vi "setArmAngles.vi"(1 "Enum":T1(ring), 2 "speed":i32, 3 "angle":i32) -> ()   [LabVIEW 2018]
uses:
  ARM angles.vi
panel:
  out "output variable":i32
  out "s2":i32
  out "s1":i32
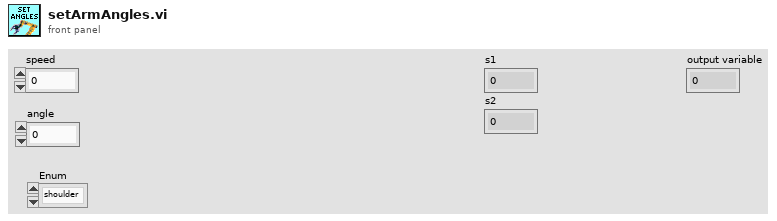
[diagram p1: front panel]
types:
  T1 = enum16{"shoulder", "elbow", "wrist", "base", "gripper"}
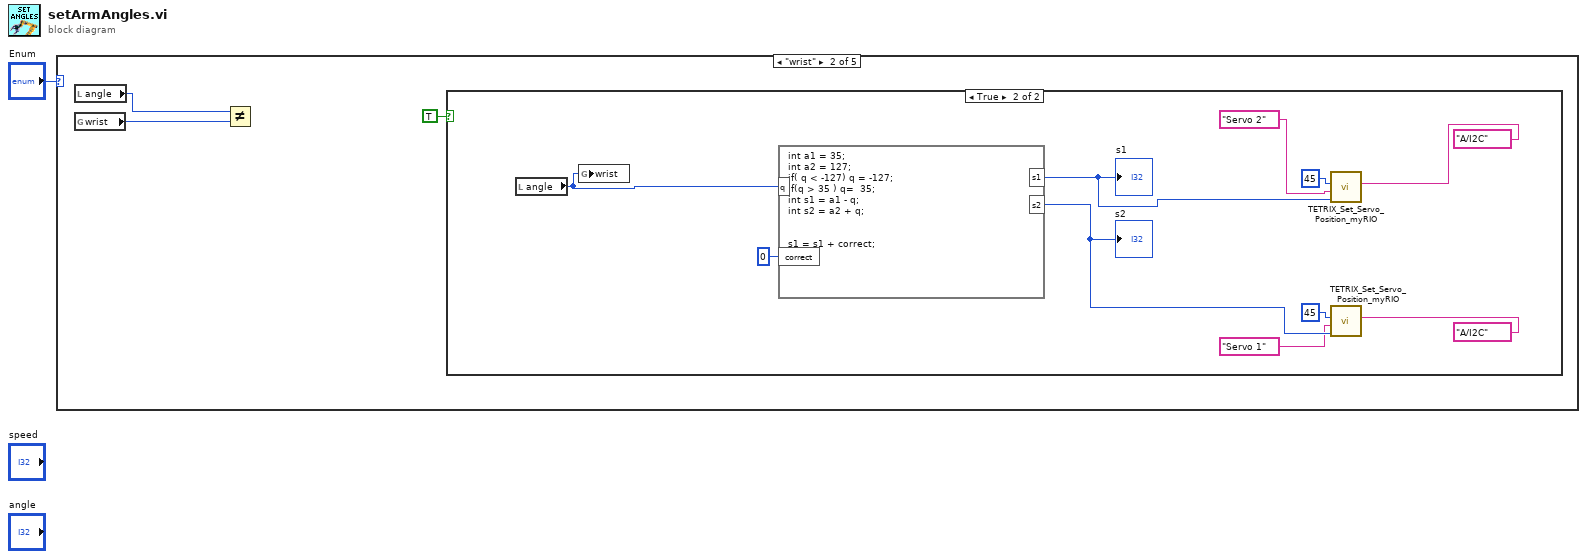
[diagram p0: block diagram]
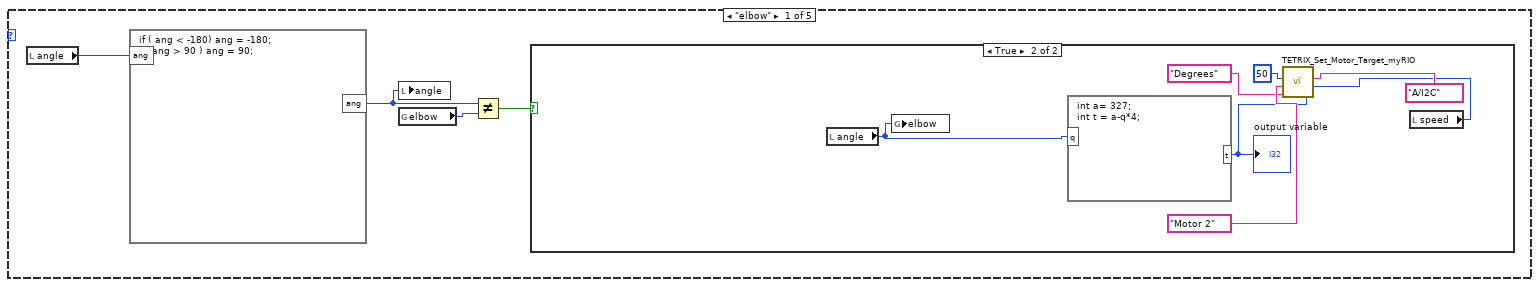
[diagram p2: hidden frame]
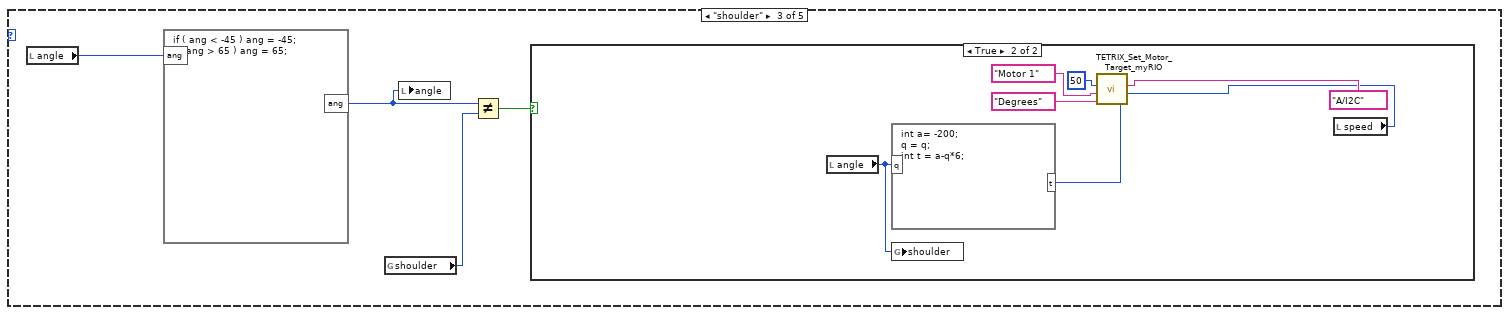
[diagram p5: hidden frame]
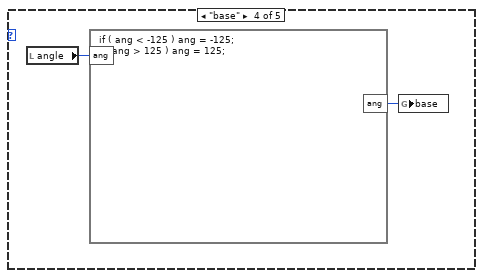
[diagram p7: hidden frame]
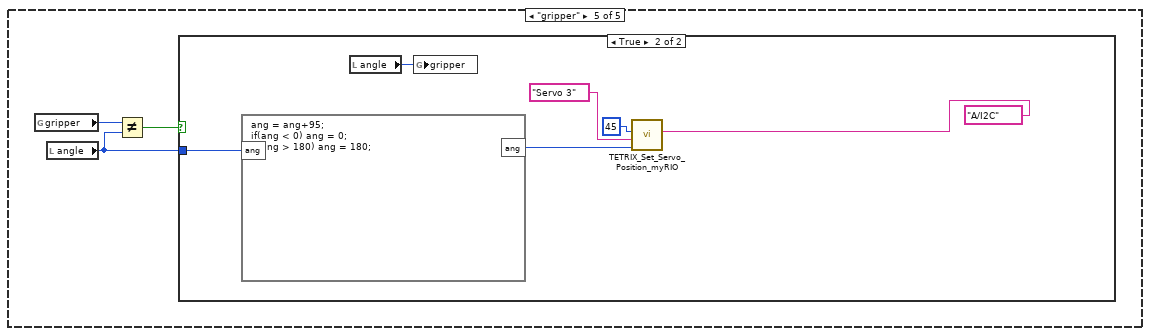
[diagram p8: hidden frame]
diagram:
  n1 = case shown="\"wrist\"" "Enum" {
    frame "elbow" {
      n2 = local read "angle"() -> (w3:i32)
      n3 = formula code="if ( ang < -180) ang = -180;\nif( ang > 90 ) ang = 90;"("ang"=w3) -> ("ang"=w2:i32)
      n4 = local write "angle"(w2) -> ()
      n5 = global read "ARM angles.vi" "elbow"() -> (w5:i32)
      n6 = Not Equal?(x=w2, y=w5) -> (x != y?=w4:bool)
      n7 = case shown="True" w4 {
        frame False {
        }
        frame True {
          n8 = local read "angle"() -> (w7:i32)
          n9 = global write "ARM angles.vi" "elbow"(w7) -> ()
          n10 = formula code="int a= 327;\nint t = a-q*4;"("q"=w7) -> ("t"=w6:i32)
          "output variable" <- w6
          n11 = local read "speed"() -> (w8:i32)
          n12 = call <vilib>:"TETRIX_Set_Motor_Target_myRIO.vi"("Motor Encoder Target"=w6, "Constant Speed (Degrees per Second)"=w8, "myRIO MXP Port A/B"=tag "A/I2C", "Encoder Units"="Degrees", "Select Channel"="Motor 2", "Controller ID#  (I2C Address)"=u8 50) -> ()  [unwired: 1 in, 1 out]
        }
      }
    }
    frame "wrist" {
      n13 = local read "angle"() -> (w14:i32)
      n14 = global read "ARM angles.vi" "wrist"() -> (w15:i32)
      n15 = Not Equal?(x=w14, y=w15) -> ()  [unwired: 1 out]
      n16 = case shown="True" TRUE {
        frame False {
        }
        frame True {
          n17 = local read "angle"() -> (w25:i32)
          n18 = global write "ARM angles.vi" "wrist"(w25) -> ()
          n19 = formula code="int a1 = 35;\nint a2 = 127;\nif( q < -127) q = -127;\nif(q > 35 ) q=  35;\nint s1 = a1 - q;\nint s2 = a2 + q;\n\n\ns1 = s1 + correct;"("q"=w25, "correct"=0 ("input variable")) -> ("s2"=w21:i32, "s1"=w20:i32)
          "s1" <- w20
          "s2" <- w21
          n20 = call <vilib>:"TETRIX_Set_Servo_Position_myRIO.vi"("myRIO MXP Port A/B"=tag "A/I2C", "Set Servo Position (0 - 180 degrees)"=w20, "Select Channel"="Servo 2", "Controller ID#  (I2C Address)"=u8 45) -> ()  [unwired: 3 in, 1 out]
          n21 = call <vilib>:"TETRIX_Set_Servo_Position_myRIO.vi"("myRIO MXP Port A/B"=tag "A/I2C", "Set Servo Position (0 - 180 degrees)"=w21, "Select Channel"="Servo 1", "Controller ID#  (I2C Address)"=u8 45) -> ()  [unwired: 3 in, 1 out]
        }
      }
    }
    frame "shoulder" {
      n22 = local read "angle"() -> (w27:i32)
      n23 = formula code="if ( ang < -45 ) ang = -45;\nif( ang > 65 ) ang = 65;"("ang"=w27) -> ("ang"=w26:i32)
      n24 = global read "ARM angles.vi" "shoulder"() -> (w29:i32)
      n25 = local write "angle"(w26) -> ()
      n26 = Not Equal?(x=w26, y=w29) -> (x != y?=w28:bool)
      n27 = case shown="True" w28 {
        frame False {
        }
        frame True {
          n28 = local read "angle"() -> (w31:i32)
          n29 = formula code="int a= -200;\nq = q;\nint t = a-q*6;"("q"=w31) -> ("t"=w30:i32)
          n30 = global write "ARM angles.vi" "shoulder"(w31) -> ()
          n31 = local read "speed"() -> (w32:i32)
          n32 = call <vilib>:"TETRIX_Set_Motor_Target_myRIO.vi"("Motor Encoder Target"=w30, "Constant Speed (Degrees per Second)"=w32, "myRIO MXP Port A/B"=tag "A/I2C", "Encoder Units"="Degrees", "Select Channel"="Motor 1", "Controller ID#  (I2C Address)"=u8 50) -> ()  [unwired: 1 in, 1 out]
        }
      }
    }
    frame "base" {
      n33 = local read "angle"() -> (w38:i32)
      n34 = formula code="if ( ang < -125 ) ang = -125;\nif( ang > 125 ) ang = 125;"("ang"=w38) -> ("ang"=w37:i32)
      n35 = global write "ARM angles.vi" "base"(w37) -> ()
    }
    frame "gripper" {
      n36 = global read "ARM angles.vi" "gripper"() -> (w41:i32)
      n37 = local read "angle"() -> (w39:i32)
      n38 = Not Equal?(x=w41, y=w39) -> (x != y?=w40:bool)
      n39 = case shown="True" w40 {
        tunnel: w39 -> [_ w47]
        frame False {
        }
        frame True {
          n40 = formula code="ang = ang+95;\nif(ang < 0) ang = 0;\nif(ang > 180) ang = 180;"("ang"=w47) -> ("ang"=w42:i32)
          n41 = local read "angle"() -> (w46:i32)
          n42 = global write "ARM angles.vi" "gripper"(w46) -> ()
          n43 = call <vilib>:"TETRIX_Set_Servo_Position_myRIO.vi"("myRIO MXP Port A/B"=tag "A/I2C", "Set Servo Position (0 - 180 degrees)"=w42, "Select Channel"="Servo 3", "Controller ID#  (I2C Address)"=u8 45) -> ()  [unwired: 3 in, 1 out]
        }
      }
    }
  }
